vi "LeyboldTurbo_Main.vi"() -> ()   [LabVIEW 2019]
doc: "Example VI to demonstrate the use of the Oerlikon Leybold TMP driver."
uses:
  <vilib>/Utility/error.llb/Error Cluster From Error Code.vi
  <vilib>/ErrorRing/Error Ring.xnode
  <instrlib>/Leybold TURBOVAC/Leybold TURBOVAC.lvlib
panel:
  out "meter_freq":cluster{dbl, dbl}(knob) caption="Frequency (Hz)" scale=0.0..700.0 scale format="%#.2f"
  in  "Tab Control":T1(tab)
  out "status_word_1":T2 caption="Status words 1"
  out "status_word_2":T2 caption="Status words 2"
  out "chart_freq":waveform(dbl)[](graph)
  out "chart_curr":waveform(dbl)[](graph)
  out "chart_temp":waveform(dbl)[](graph)
  in  "VISA2":refnum<visa-resource-name>="COM43"
  in  "VISA1":refnum<visa-resource-name>="COM44" caption="VISA"
  out "status_cont_2":bool caption="Control status"
  in  "operate_2":bool caption="Operate"
  out "temp_2":i32 caption="Temperature"
  out "current_2":dbl
  out "freq_2":u16
  out "current_1":dbl caption="Current"
  out "freq_1":u16 caption="Frequency"
  in  "SN":string[](array[string])=["240804202", "240804204"]
  out "temp_1":i32 caption="Temperature"
  out "time_meas":timestamp caption="Last update" format="%<%Y-%m-%d %H:%M:%S>T"
  out "status_cont_1":bool caption="Control status"
  in  "interval":u32=1000 caption="Interval"
  in  "remote_cont":bool caption="Remote Control"
  in  "operate_1":bool caption="Operate"
  in  "stop":bool
  # "IVC Turbo Pumps"
  # "Leybold TURBOVAC 1350iR + TURBO.DRIVE 500e"
  # "Turbo #1"
  # "Turbo #2"
  # "ms"
  # "Turbo #1"
  # "Turbo #2"
  # "Hz"
  # "Hz"
  # "A"
  # "A"
  # "°C"
  # "°C"
  # "Turbo #1\nTurbo #2"
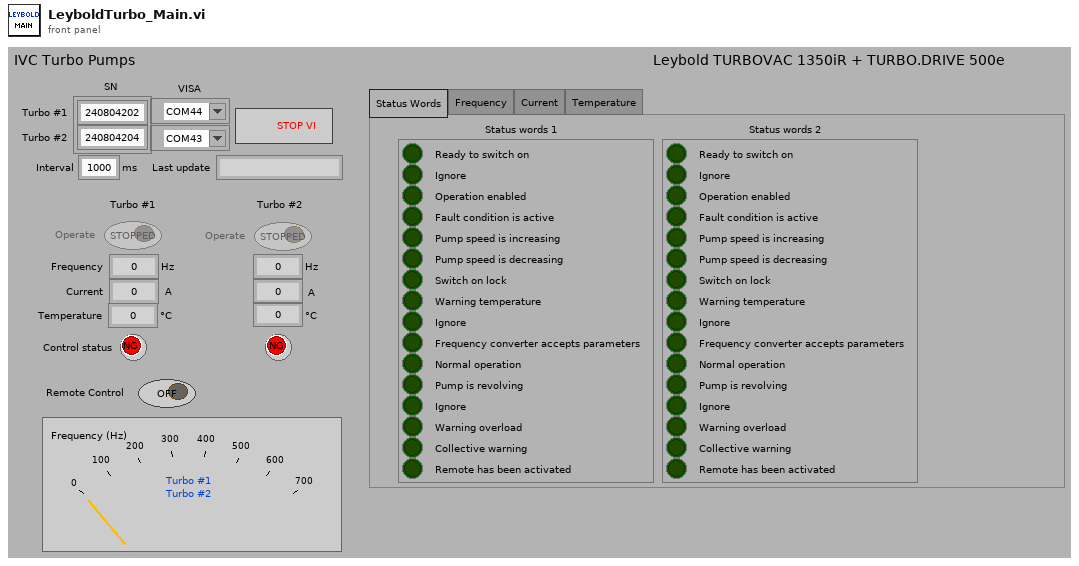
[diagram p1: front panel]
types:
  T1 = enum32{"Status Words", "Frequency", "Current", "Temperature"}
  T2 = cluster{"Ready to switch on":bool, "Ignore":bool, "Operation enabled":bool, "Fault condition is active":bool, "Pump speed is increasing":bool, "Pump speed is decreasing":bool, "Switch on lock":bool, "Warning temperature":bool, "Ignore":bool, "Frequency converter accepts parameters":bool, "Normal operation":bool, "Pump is revolving":bool, "Ignore":bool, "Warning overload":bool, "Collective warning":bool, "Remote has been activated":bool}
  T3 = enum8{"Enabled", "Disabled", "Disabled and Grayed Out"}
  T4 = typedef "Leybold TURBOVAC.lvlib/Device Parameters Indicator.ctl" = cluster{"Length of data block":u8, "Converter address":u8, "Converter type":T5, "PZD1":u16, "PZD2":u16}
  T5 = typedef "Leybold TURBOVAC.lvlib/Converter Type Indicator.ctl" = u16
  T6 = cluster{"Actual stator frequency [Hz]":u16, "Converter temperature [°C]":u16, "Motor current [A]":dbl, "Intermediate circuit voltage Uzk [V]":dbl}
  T7 = cluster{"Actual stator frequency [Hz]":u16, "Actual stator frequency [Hz]":u16}
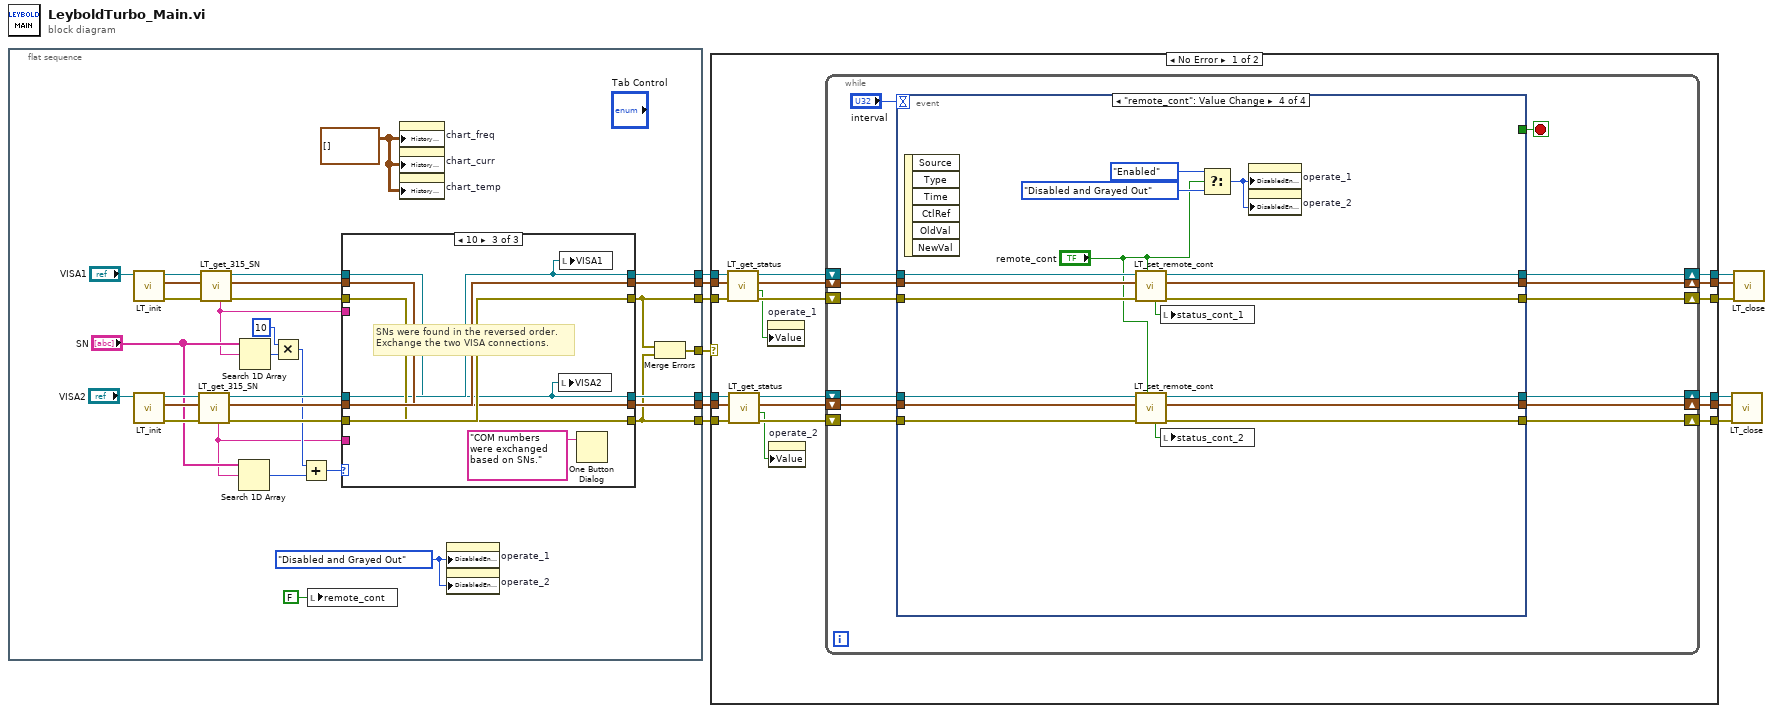
[diagram p0: block diagram]
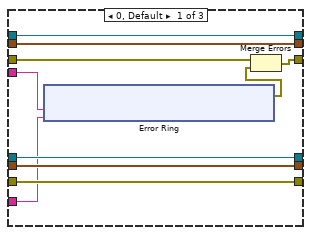
[diagram p2: hidden frame]
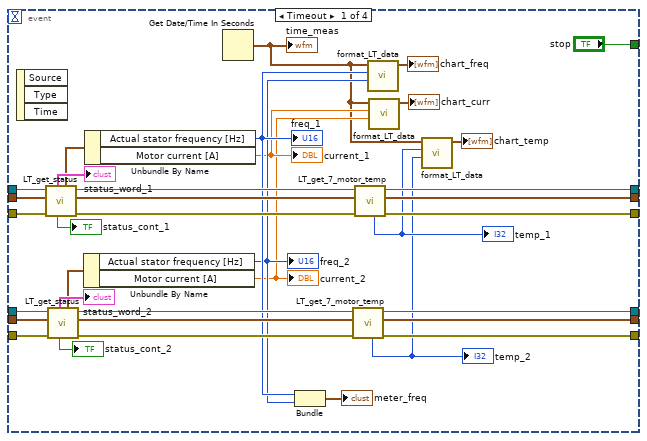
[diagram p4: hidden frame]
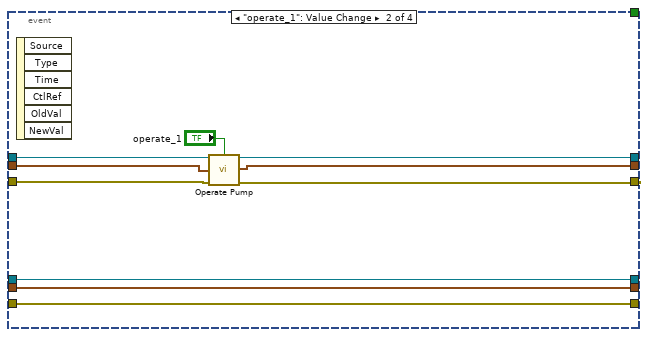
[diagram p5: hidden frame]
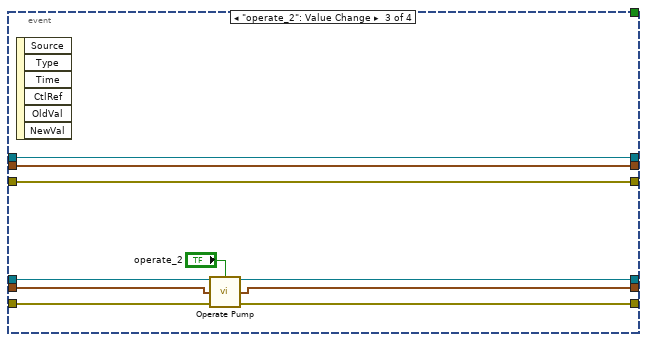
[diagram p6: hidden frame]
diagram:
  n1 = flat-sequence {
    tunnel: [w34] -> w10
    tunnel: [w33] -> w9
    tunnel: [w29] -> w8
    tunnel: [w28] -> w7
    tunnel: [w21] -> w6
    tunnel: [w20] -> w5
    tunnel: [w19] -> w4
    frame #0 {
      w14 = T3."Disabled and Grayed Out" ("Disabled")
      w16 = waveform(dbl)[][] [] ("History Data")
      n2 = call "LT_init.vi"("VISA in"="VISA1") -> ("error out"=w42:errorcluster, "dev_param_out"=w43:T4, "VISA out"=w44:refnum<visa-resource-name>)  [unwired: 7 in, 1 out]
      n3 = call "LT_init.vi"("VISA in"="VISA2") -> ("error out"=w39:errorcluster, "dev_param_out"=w40:T4, "VISA out"=w41:refnum<visa-resource-name>)  [unwired: 7 in, 1 out]
      n4 = call "LT_get_315_SN.vi"("error in"=w39, "dev_param_in"=w40, "VISA in"=w41) -> ("error out"=w30:errorcluster, "dev_param_out"=w31:T4, "VISA out"=w32:refnum<visa-resource-name>, "SN_converter"=w17:string)  [unwired: 5 in]
      n5 = call "LT_get_315_SN.vi"("error in"=w42, "dev_param_in"=w43, "VISA in"=w44) -> ("error out"=w35:errorcluster, "dev_param_out"=w36:T4, "VISA out"=w37:refnum<visa-resource-name>, "SN_converter"=w18:string)  [unwired: 5 in]
      n6 = Search 1D Array(1D array="SN", element=w17) -> (index of element=w23:i32)  [unwired: 1 in]
      n7 = Search 1D Array(1D array="SN", element=w18) -> (index of element=w26:i32)  [unwired: 1 in]
      n8 = Multiply(x=10, y=w26) -> (x*y=w24:i32)
      n9 = Add(x=w24, y=w23) -> (x+y=w22:i32)
      n10 = local write "remote_cont"(FALSE ("remote_cont")) -> ()
      n11 = case shown="10" w22 {
        tunnel: w37 -> [w55 w65 w71]
        tunnel: w36 -> [w54 w68 w74]
        tunnel: w35 -> [w50 w69 w73]
        tunnel: [w49 w69 w76] -> w21
        tunnel: [w54 w68 w75] -> w34
        tunnel: [w55 w65 w72] -> w33
        tunnel: w32 -> [w53 w64 w72]
        tunnel: w31 -> [w52 w67 w75]
        tunnel: w30 -> [w51 w66 w76]
        tunnel: [w53 w64 w71] -> w29
        tunnel: [w52 w67 w74] -> w28
        tunnel: [w51 w66 w73] -> w20
        tunnel: w18 -> [w47 _ _]
        tunnel: w17 -> [w46 _ _]
        frame 0, Default {
          n12 = xnode "Error Ring"("parameter 0"=w47, "parameter 1"=w46) -> ("error out"=w48:errorcluster)
          n13 = Merge Errors(w50, w48) -> (w49:errorcluster)
        }
        frame 1 {
          # "SNs were found in the normal order."
        }
        frame 10 {
          # "SNs were found in the reversed order.\nExchange the two VISA connections."
          n14 = local write "VISA2"(w71) -> ()
          n15 = local write "VISA1"(w72) -> ()
          n16 = One Button Dialog(message="COM numbers were exchanged based on SNs.") -> ()  [unwired: 1 in, 1 out]
        }
      }
      n17 = property on="chart_freq" class="WFChart (strict)"("History Data"=w16) -> ()  [unwired: 2 in, 2 out]
      n18 = property on="chart_curr" class="WFChart (strict)"("History Data"=w16) -> ()  [unwired: 2 in, 2 out]
      n19 = property on="chart_temp" class="WFChart (strict)"("History Data"=w16) -> ()  [unwired: 2 in, 2 out]
      n20 = property on="operate_1" class="Bool (strict)"("DisabledEnum"=w14) -> ()  [unwired: 2 in, 2 out]
      n21 = property on="operate_2" class="Bool (strict)"("DisabledEnum"=w14) -> ()  [unwired: 2 in, 2 out]
      n22 = Merge Errors(w21, w20) -> (w19:errorcluster)
    }
  }
  n23 = case shown="No Error" w4 {
    tunnel: w9 -> [w89 w189]
    tunnel: w10 -> [w88 w190]
    tunnel: [w96 w189] -> w13
    tunnel: [w95 w190] -> w11
    tunnel: [w94 w188] -> w12
    tunnel: w8 -> [w86 w187]
    tunnel: w7 -> [w85 w185]
    tunnel: w5 -> [w84 w186]
    tunnel: w6 -> [w87 w188]
    tunnel: [w80 w187] -> w3
    tunnel: [w78 w186] -> w2
    tunnel: [w79 w185] -> w1
    frame No Error {
      n24 = call "LT_get_status.vi"("error in"=w87, "dev_param_in"=w88, "VISA in"=w89) -> ("error out"=w92:errorcluster, "op_enabled"=w90:bool, "dev_param_out"=w91:T4, "VISA out"=w93:refnum<visa-resource-name>)  [unwired: 1 in, 4 out]
      n25 = call "LT_get_status.vi"("error in"=w84, "dev_param_in"=w85, "VISA in"=w86) -> ("error out"=w81:errorcluster, "op_enabled"=w77:bool, "dev_param_out"=w82:T4, "VISA out"=w83:refnum<visa-resource-name>)  [unwired: 1 in, 4 out]
      n26 = property on="operate_1" class="Bool (strict)"("Value"=w90) -> ()  [unwired: 2 in, 2 out]
      n27 = property on="operate_2" class="Bool (strict)"("Value"=w77) -> ()  [unwired: 2 in, 2 out]
      n28 = while {
        shift-right: [w105] -> w95
        shift-left: w91 -> [w106]
        shift-right: [w104] -> w94
        shift-left: w92 -> [w108]
        shift-right: [w109] -> w96
        shift-left: w93 -> [w107]
        shift-right: [w99] -> w80
        shift-left: w83 -> [w102]
        shift-right: [w98] -> w79
        shift-left: w82 -> [w100]
        shift-right: [w97] -> w78
        shift-left: w81 -> [w101]
        stop <- w110 stop-if-true
        n29 = event shown="[3] \"remote_cont\": Value Change" {
          selector: _ -> [_ _ _ _]
          dyn-events: _ -> [_ _ _ _]
          timeout: "interval" -> [_ _ _ _]
          tunnel: ["stop" _ _ _] -> w110
          tunnel: [w139 w152 w159 w180] -> w109
          tunnel: w108 -> [w144 w153 w157 w183]
          tunnel: w107 -> [w145 w155 w159 w182]
          tunnel: w106 -> [w143 w154 w158 w181]
          tunnel: [w137 w151 w158 w179] -> w105
          tunnel: [w135 w150 w157 w184] -> w104
          tunnel: w102 -> [w134 w149 w165 w178]
          tunnel: w101 -> [w133 w147 w164 w177]
          tunnel: w100 -> [w132 w148 w163 w173]
          tunnel: [w128 w149 w162 w174] -> w99
          tunnel: [w127 w148 w160 w175] -> w98
          tunnel: [w126 w147 w161 w176] -> w97
          event Timeout {
            n30 = event-data() -> ()  [unwired: 1 in, 3 out]
            n31 = call "LT_get_status.vi"("error in"=w144, "dev_param_in"=w143, "VISA in"=w145) -> ("error out"=w136:errorcluster, "dev_param_out"=w138:T4, "VISA out"=w140:refnum<visa-resource-name>, "Status values"=w125:T6, "status_cont"=→"status_cont_1":bool, "Status word"=→"status_word_1":T2)  [unwired: 1 in, 2 out]
            n32 = call "LT_get_status.vi"("error in"=w133, "dev_param_in"=w132, "VISA in"=w134) -> ("error out"=w130:errorcluster, "dev_param_out"=w129:T4, "VISA out"=w131:refnum<visa-resource-name>, "Status values"=w123:T6, "status_cont"=→"status_cont_2":bool, "Status word"=→"status_word_2":T2)  [unwired: 1 in, 2 out]
            n33 = Unbundle By Name(w123) -> ("Actual stator frequency [Hz]"=w119:u16, "Motor current [A]"=w116:dbl)
            "freq_2" <- w119
            "current_2" <- w116
            n34 = Unbundle By Name(w125) -> ("Actual stator frequency [Hz]"=w120:u16, "Motor current [A]"=w117:dbl)
            "freq_1" <- w120
            "current_1" <- w117
            n35 = Get Date/Time In Seconds() -> (seconds since 1Jan1904=w112:timestamp)
            "time_meas" <- w112
            n36 = Bundle("Actual stator frequency [Hz]"=w120, "Actual stator frequency [Hz]"=w119) -> (→"meter_freq":T7)  [unwired: 1 in]
            n37 = call "LT_get_7_motor_temp.vi"("error in"=w130, "dev_param_in"=w129, "VISA in"=w131) -> ("error out"=w126:errorcluster, "dev_param_out"=w127:T4, "VISA out"=w128:refnum<visa-resource-name>, "temp"=w113:i32)  [unwired: 5 in]
            "temp_2" <- w113
            n38 = call "LT_get_7_motor_temp.vi"("error in"=w136, "dev_param_in"=w138, "VISA in"=w140) -> ("error out"=w135:errorcluster, "dev_param_out"=w137:T4, "VISA out"=w139:refnum<visa-resource-name>, "temp"=w114:i32)  [unwired: 5 in]
            "temp_1" <- w114
            n39 = call "format_LT_data.vi"("value_2"=w119, "value_1"=w120, "time"=w112) -> ("waveform_array"=→"chart_freq":waveform(dbl)[])  [unwired: 8 in]
            n40 = call "format_LT_data.vi"("value_2"=w116, "value_1"=w117, "time"=w112) -> ("waveform_array"=→"chart_curr":waveform(dbl)[])  [unwired: 8 in]
            n41 = call "format_LT_data.vi"("value_2"=w113, "value_1"=w114, "time"=w112) -> ("waveform_array"=→"chart_temp":waveform(dbl)[])  [unwired: 8 in]
          }
          event "operate_1": Value Change {
            n42 = event-data() -> ()  [unwired: 1 in, 6 out]
            n43 = call <instrlib>:"Operate Pump.vi"("VISA resource name"=w155, "Operate pump (F: off)"="operate_1", "Device parameters"=w154, "error in (no error)"=w153) -> ("VISA resource name out"=w152:refnum<visa-resource-name>, "Device parameters out"=w151:T4, "error out"=w150:errorcluster)  [unwired: 9 in]
          }
          event "operate_2": Value Change {
            n44 = event-data() -> ()  [unwired: 1 in, 6 out]
            n45 = call <instrlib>:"Operate Pump.vi"("VISA resource name"=w165, "Operate pump (F: off)"="operate_2", "Device parameters"=w163, "error in (no error)"=w164) -> ("VISA resource name out"=w162:refnum<visa-resource-name>, "Device parameters out"=w160:T4, "error out"=w161:errorcluster)  [unwired: 9 in]
          }
          event "remote_cont": Value Change {
            n46 = event-data() -> ()  [unwired: 1 in, 6 out]
            n47 = call "LT_set_remote_cont.vi"("remote_cont"="remote_cont", "error in"=w183, "dev_param_in"=w181, "VISA in"=w182) -> ("error out"=w184:errorcluster, "dev_param_out"=w179:T4, "VISA out"=w180:refnum<visa-resource-name>, "status"=w172:bool)  [unwired: 4 in]
            n48 = call "LT_set_remote_cont.vi"("remote_cont"="remote_cont", "error in"=w177, "dev_param_in"=w173, "VISA in"=w178) -> ("error out"=w176:errorcluster, "dev_param_out"=w175:T4, "VISA out"=w174:refnum<visa-resource-name>, "status"=w171:bool)  [unwired: 4 in]
            n49 = local write "status_cont_1"(w172) -> ()
            n50 = local write "status_cont_2"(w171) -> ()
            n51 = Select(t=T3."Enabled" ("Disabled"), s="remote_cont", f=T3."Disabled and Grayed Out" ("Disabled")) -> (s? t:f=w170:T3)
            n52 = property on="operate_1" class="Bool (strict)"("DisabledEnum"=w170) -> ()  [unwired: 2 in, 2 out]
            n53 = property on="operate_2" class="Bool (strict)"("DisabledEnum"=w170) -> ()  [unwired: 2 in, 2 out]
          }
        }
      }
    }
    frame Error {
    }
  }
  n54 = call "LT_close.vi"("error in"=w2, "dev_param_in"=w1, "VISA in"=w3) -> ()  [unwired: 9 in]
  n55 = call "LT_close.vi"("error in"=w12, "dev_param_in"=w11, "VISA in"=w13) -> ()  [unwired: 9 in]
